vi "Select_Files.vi"(8 "error in":errorcluster, 10 "Select Files":string[](array[string])) -> (0 "error out":errorcluster, 1 "Selected External File Paths":path[](array[path]), 2 "Selected LV Files":string[](array[string]))   [LabVIEW 2013]
panel:
  in  "External Files (select by browsing)":path[](array[path])
  in  "Okay":bool
  in  "LV Files (Select with X box)":cluster{"File":string, "Boolean":bool}[](array[cluster])
  # "Select Files to include in module from below:"
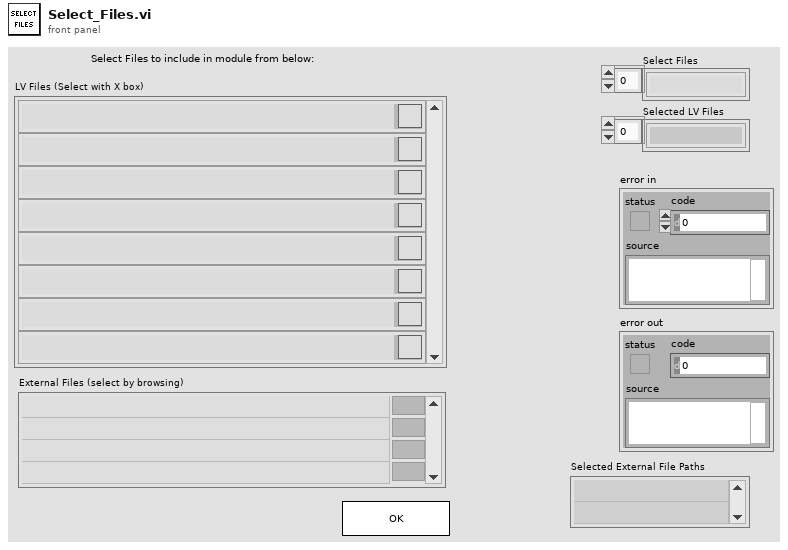
[diagram p1: front panel]
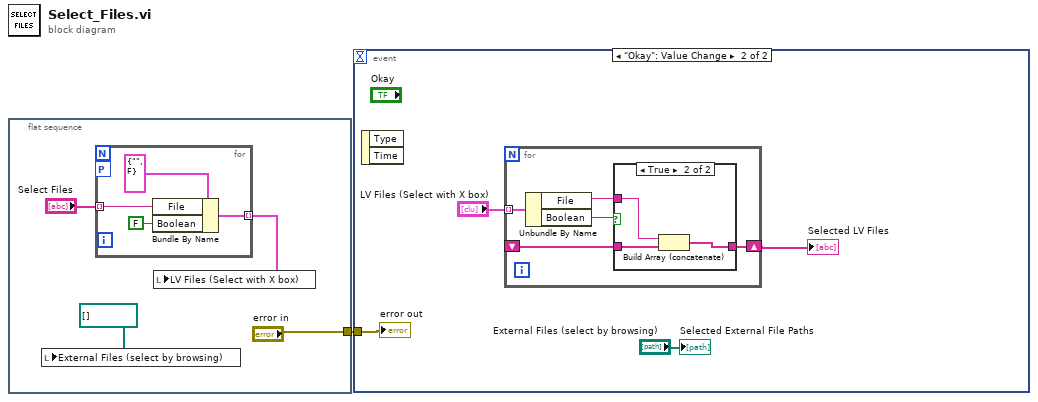
[diagram p0: block diagram]
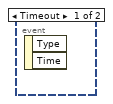
[diagram p2: hidden frame]
diagram:
  n1 = flat-sequence {
    tunnel: ["error in"] -> w1
    frame #0 {
      n2 = local write "External Files (select by browsing)"(path[] [] ("External Files")) -> ()
      n3 = for {
        workers-P: _ -> [_]
        tunnel: "Select Files" -> [w7] mode=indexing
        tunnel: [w6] -> w3 mode=indexing
        n4 = Bundle By Name(cluster=cluster{"File":string, "Boolean":bool} {"File"="", "Boolean"=FALSE} ("Files"), "File"=w7, "Boolean"=FALSE) -> (w6:cluster{"File":string, "Boolean":bool})
      }
      n5 = local write "LV Files (Select with X box)"(w3) -> ()
    }
  }
  n6 = event shown="[1] \"Okay\": Value Change" {
    selector: _ -> [_ _]
    dyn-events: _ -> [_ _]
    timeout: _ -> [_ _]
    tunnel: w1 -> [_ w12]
    event Timeout {
      n7 = event-data() -> ()  [unwired: 1 in, 2 out]
    }
    event "Okay": Value Change {
      n8 = event-data() -> ()  [unwired: 1 in, 2 out]
      n9 = for {
        shift-right: [w18] -> w11
        shift-left: _ -> [w14]
        tunnel: "LV Files (Select with X box)" -> [w17] mode=indexing
        n10 = Unbundle By Name(w17) -> ("File"=w16:string, "Boolean"=w15:bool)
        n11 = case shown="True" w15 {
          tunnel: [w19 w22] -> w18
          tunnel: w16 -> [_ w21]
          tunnel: w14 -> [w19 w20]
          frame False {
          }
          frame True {
            n12 = Build Array (concatenate)(w21, w20) -> (w22:string[])
          }
        }
      }
      "Selected LV Files" <- w11
      "error out" <- w12
      "Selected External File Paths" <- "External Files (select by browsing)"
    }
  }
